vi "Gray Morphological Reconstruction.vi"() -> ()   [LabVIEW 2014]
doc: "This example demonstrates a grayscale morphological reconstruction. The example reconstructs the image using the chosen ROI as a marker."
uses:
  <vilib>/vision/NI_Vision_Development_Module.lvlib
panel:
  in  "Operation":enum16{"Dilate", "Erode"}(ring)
  out "Reconstructed Image":T1(plugin-control)
  out "Image":T1(plugin-control)
  in  "Stop":bool
  # "Overview: Demonstrate the use of the Gray Morphological Reconstruction feature of Vision Development Module.\nRequirements: Vision Development Module.\nInstructions:\n1. Run the VI.\n2. Draw an ROI in the source Image. The objects at the boundary of the ROI gets reconstructed. Press the <Ctrl> key to select multiple ROIs.\n3. Modify Operation."
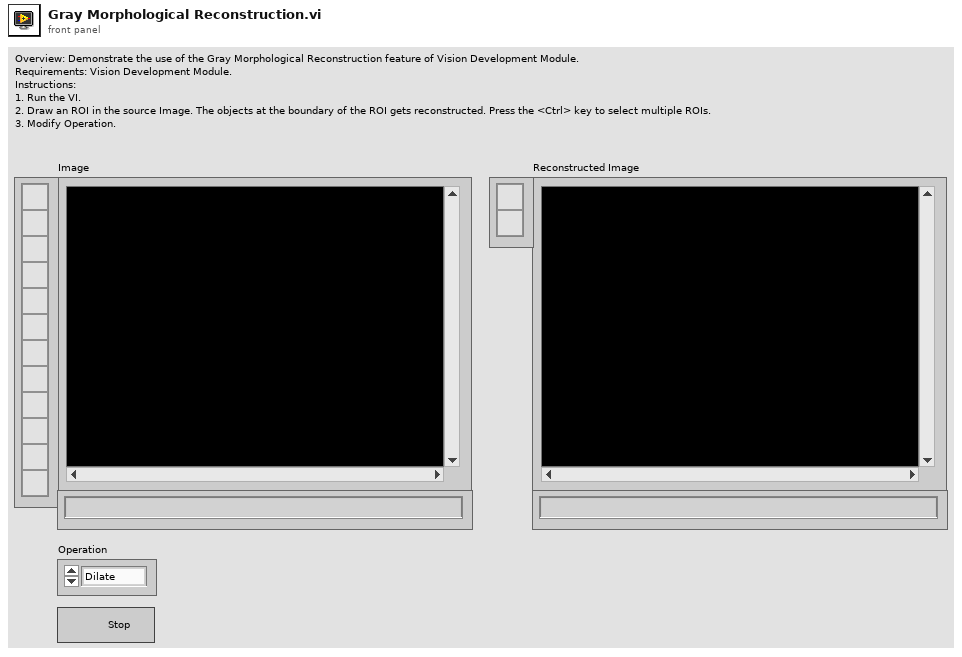
[diagram p1: front panel]
types:
  T1 = typedef "IMAQ Image.ctl" = refnum<image>
  T2 = typedef "Image Type" = u32
  T3 = cluster{"Global Rectangle":i32[], "Contours":cluster{"Contour Type":u32, "ROI Type":u32, "Points":i32[]}[]}
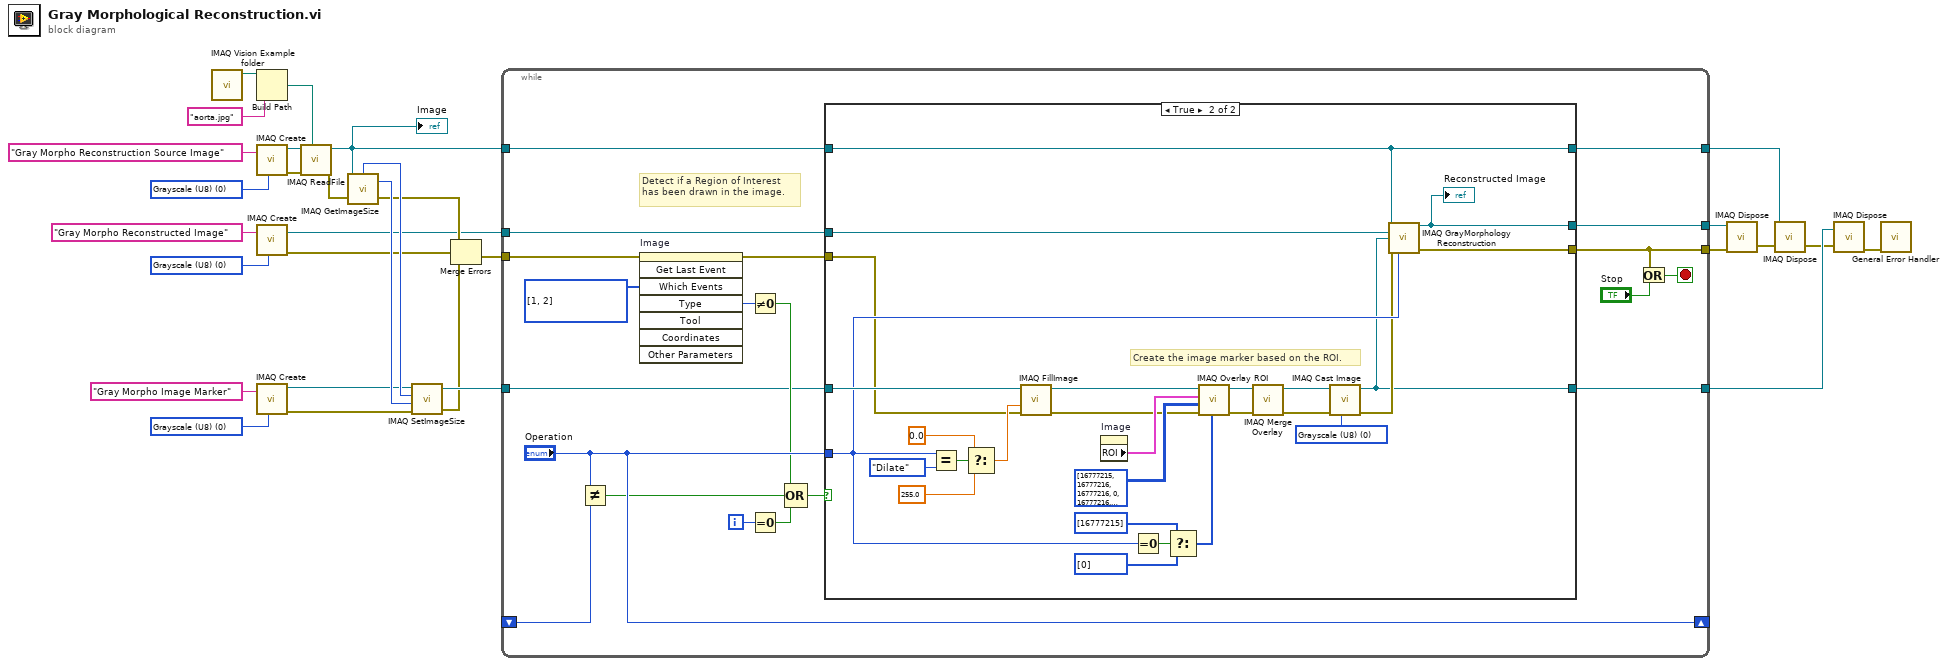
[diagram p0: block diagram]
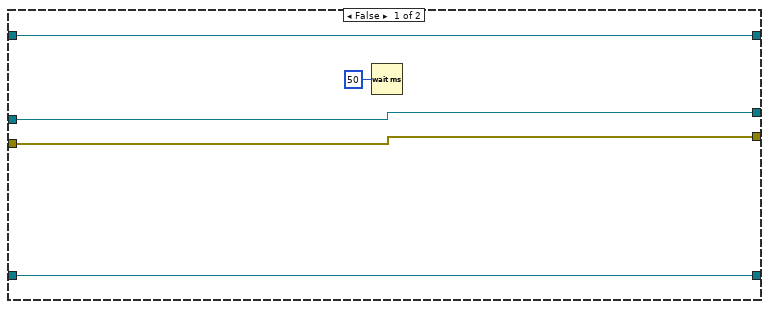
[diagram p2: hidden frame]
diagram:
  w20 = T2 0 items=["Grayscale (U8)", "Grayscale (I16)", "Grayscale (SGL)", "Complex (CSG)", "RGB (U32)", "HSL (U32)", "RGB (U64)", "Grayscale (U16)"] ("Image Type")
  w22 = T2 0 items=["Grayscale (U8)", "Grayscale (I16)", "Grayscale (SGL)", "Complex (CSG)", "RGB (U32)", "HSL (U32)", "RGB (U64)", "Grayscale (U16)"] ("Image Type")
  w23 = T2 0 items=["Grayscale (U8)", "Grayscale (I16)", "Grayscale (SGL)", "Complex (CSG)", "RGB (U32)", "HSL (U32)", "RGB (U64)", "Grayscale (U16)"] ("Image Type")
  n1 = call "IMAQ Vision Example folder.vi"() -> ("Example Image Path"=w29:path)  [unwired: 11 in]
  n2 = Build Path(base path=w29, name or relative path="aorta.jpg") -> (appended path=w4:path)
  n3 = call "IMAQ Create"("Image Name"="Gray Morpho Reconstruction Source Image", "Image Type"=w22) -> ("New Image"=w26:T1, "error out"=w17:errorcluster)  [unwired: 2 in, 1 out]
  n4 = call "IMAQ Create"("Image Name"="Gray Morpho Reconstructed Image", "Image Type"=w23) -> ("New Image"=w5:T1, "error out"=w16:errorcluster)  [unwired: 2 in, 1 out]
  n5 = call "IMAQ Create"("Image Name"="Gray Morpho Image Marker", "Image Type"=w20) -> ("New Image"=w10:T1, "error out"=w8:errorcluster)  [unwired: 2 in, 1 out]
  n6 = call "IMAQ ReadFile"("File Path"=w4, "error in (no error)"=w17, "Image"=w26) -> ("error out"=w11:errorcluster, "Image Out"=w12:T1)  [unwired: 2 in, 5 out]
  "Image" <- w12
  n7 = call "IMAQ GetImageSize"("Image"=w12, "error in (no error)"=w11) -> ("Y Resolution"=w18:i32, "X Resolution"=w19:i32, "error out"=w14:errorcluster)  [unwired: 2 out]
  n8 = call "IMAQ SetImageSize"("error in (no error)"=w8, "Y Resolution"=w18, "X Resolution"=w19, "Image"=w10) -> ("error out"=w7:errorcluster, "Image Out"=w9:T1)  [unwired: 1 out]
  n9 = Merge Errors(w14, w16, w7) -> (w6:errorcluster)
  n10 = while {
    tunnel: w12 -> [w50]
    tunnel: w5 -> [w39]
    tunnel: [w37] -> w25
    tunnel: [w38] -> w24
    tunnel: w9 -> [w40]
    shift-right: ["Operation"] -> _
    shift-left: _ -> [w49]
    tunnel: w6 -> [w45]
    tunnel: [w33] -> w15
    tunnel: [w36] -> w13
    i -> [w42]
    stop <- w31 stop-if-true
    w46 = i32[] [1, 2] items=["No Event"=0, "Click Event"=1, "Draw Event"=2, "Size Event"=4, "Scroll Event"=5, "Double Click Event"=8] ("Which Events")
    # "Detect if a Region of Interest has been drawn in the image."
    n11 = Not Equal?(x="Operation", y=w49) -> (x != y?=w35:bool)
    n12 = invoke on="Image" class="ImageControl" method="Get Last Event"(error in=w45, "Which Events"=w46) -> (error out=w44:errorcluster, "Type"=w47:i32)  [unwired: 6 in, 6 out]
    n13 = Not Equal To 0?(x=w47) -> (x != 0?=w43:bool)
    n14 = Equal To 0?(x=w42) -> (x = 0?=w34:bool)
    n15 = Compound Arithmetic op=OR(w43, w35, w34) -> (w41:bool)
    n16 = case shown="True" w41 {
      tunnel: w50 -> [w53 w59]
      tunnel: w39 -> [w52 w73]
      tunnel: w40 -> [w51 w72]
      tunnel: "Operation" -> [_ w71]
      tunnel: w44 -> [w55 w60]
      tunnel: [w55 w68] -> w33
      tunnel: [w53 w59] -> w38
      tunnel: [w52 w58] -> w37
      tunnel: [w51 w56] -> w36
      frame False {
        n17 = Wait (ms)(milliseconds to wait=u32 50) -> ()  [unwired: 1 out]
      }
      frame True {
        w81 = T2 0 items=["Grayscale (U8)", "Grayscale (I16)", "Grayscale (SGL)", "Complex (CSG)", "RGB (U32)", "HSL (U32)", "RGB (U64)", "Grayscale (U16)"] ("Image Type")
        # "Create the image marker based on the ROI."
        n18 = Equal?(x=w71, y=enum16{"Dilate", "Erode"}."Dilate" ("Operation")) -> (x = y?=w76:bool)
        n19 = Select(t=sgl 0.0 ("Pixel Value (U8, U16, I16, Float)"), s=w76, f=sgl 255.0 ("Pixel Value (U8, U16, I16, Float)")) -> (s? t:f=w62:sgl)
        n20 = call "IMAQ FillImage"("error in (no error)"=w60, "Pixel Value (U8, U16, I16, Float)"=w62, "Image"=w72) -> ("error out"=w61:errorcluster, "Image Out"=w57:T1)  [unwired: 4 in, 3 out]
        n21 = property on="Image" class="ImageControl"() -> ("ROI"=w69:T3)  [unwired: 2 in, 2 out]
        n22 = Equal To 0?(x=w71) -> (x = 0?=w79:bool)
        n23 = Select(t=u32[] [16777215] ("Colors (Green)"), s=w79, f=u32[] [0] ("Colors (Green)")) -> (s? t:f=w75:u32[])
        n24 = call "IMAQ Overlay ROI"("Colors (Green)"=w75, "error in (no error)"=w61, "Point Symbol"=u32[][] [[16777215, 16777216, 16777216, 0, 16777216, 16777216, 16777216], [16777216, 16777216, 16777216, 0, 16777216, 16777216, 16777216], [16777216, 16777216, 16777216, 0, 16777216, 16777216, 16777216], [0, 0, 0, 16777216, 0, 0, 0], [16777216, 16777216, 16777216, 0, 16777216, 16777216, 16777216], [16777216, 16777216, 16777216, 0, 16777216, 16777216, 16777216], [16777216, 16777216, 16777216, 0, 16777216, 16777216, 16777216]], "ROI Descriptor"=w69, "Image"=w57) -> ("error out"=w67:errorcluster, "Image Out"=w82:T1)  [unwired: 1 in, 4 out]
        n25 = call "IMAQ Merge Overlay"("error in (no error)"=w67, "Image Src"=w82) -> ("error out"=w66:errorcluster, "Image Dst Out"=w80:T1)  [unwired: 3 in, 5 out]
        n26 = call "IMAQ Cast Image"("Image Type"=w81, "error in (no error)"=w66, "Image Src"=w80) -> ("error out"=w65:errorcluster, "Image Dst Out"=w56:T1)  [unwired: 3 in, 4 out]
        n27 = call "IMAQ GrayMorphology Reconstruction"("Image Src"=w59, "Image Dst"=w73, "Image Marker"=w56, "error in (no error)"=w65, "Operation"=w71) -> ("Image Dst Out"=w58:T1, "error out"=w68:errorcluster)  [unwired: 3 in, 6 out]
        "Reconstructed Image" <- w58
      }
    }
    n28 = Or(x=w33, y="Stop") -> (x .or. y?=w31:bool)
  }
  n29 = call "IMAQ Dispose"("Image"=w25, "error in (no error)"=w15) -> ("error out"=w3:errorcluster)  [unwired: 1 in, 3 out]
  n30 = call "IMAQ Dispose"("Image"=w24, "error in (no error)"=w3) -> ("error out"=w2:errorcluster)  [unwired: 1 in, 3 out]
  n31 = call "IMAQ Dispose"("Image"=w13, "error in (no error)"=w2) -> ("error out"=w1:errorcluster)  [unwired: 1 in, 3 out]
  n32 = call <vilib>:"General Error Handler.vi"("error in (no error)"=w1) -> ()  [unwired: 10 in, 5 out]
